vi "Get Data.vi"(8 "error in (no error)":errorcluster, 11 "DataGrid.lvlib:Abstract EVENT.lvclass":refnum<class "Abstract EVENT.lvclass">) -> (0 "error out":errorcluster, 1 "column":i32, 2 "row":i32, 3 "cell value":string)   [LabVIEW 2013, in "DataGrid.lvlib" / "CellDirtyStateChanged.lvclass"]
doc: "Converts the class data for cellValue into individual components of the grid"
uses:
  CellDirtyStateChanged.lvclass
  Abstract EVENT/Abstract EVENT.lvclass
  CellDirtyStateChanged.lvclass/CellDirtyStateChanged.ctl
  Read cell value.vi
  Read column.vi
  Read row.vi
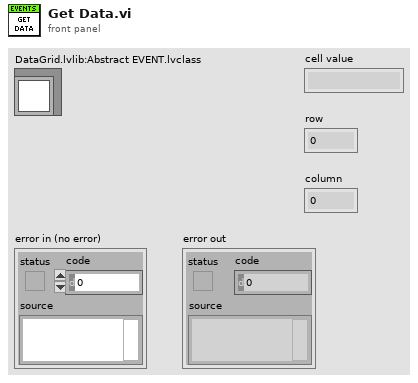
[diagram p1: front panel]
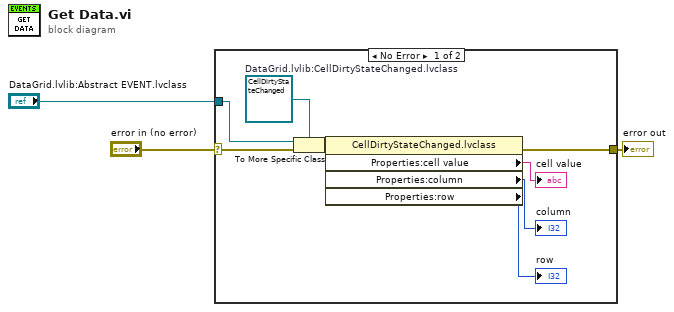
[diagram p0: block diagram]
diagram:
  n1 = case shown="No Error" "error in (no error)" {
    selector: "error in (no error)" -> [w6 w13]
    tunnel: [w12 w13] -> w2
    tunnel: "DataGrid.lvlib:Abstract EVENT.lvclass" -> [w8 _]
    frame No Error {
      w4 = refnum<class "CellDirtyStateChanged.lvclass"> refnum  # DataGrid.lvlib:CellDirtyStateChanged.lvclass
      n2 = To More Specific Class(target class=w4, reference=w8, error in=w6) -> (specific class reference=w7:refnum<class "CellDirtyStateChanged.lvclass">, error out=w5:errorcluster)
      n3 = property class="CellDirtyStateChanged.lvclass"(reference=w7, error in=w5) -> (error out=w12:errorcluster, "Properties:cell value"=→"cell value":string, "Properties:column"=→"column":i32, "Properties:row"=→"row":i32)  [unwired: 1 out]
    }
    frame Error {
    }
  }
  "error out" <- w2
